vi "End Transaction.vi"(8 "error in (no error)":errorcluster, 11 "SqlMapper in":refnum<class "SqlMapper.lvclass">) -> (0 "error out":errorcluster, 3 "SqlMapper out":refnum<class "SqlMapper.lvclass">)   [LabVIEW 2020, in "ORM.lvlib" / "SqlMapper.lvclass"]
uses:
  SqlMapper.lvclass
  SqlMapper.lvclass/SqlMapper.ctl
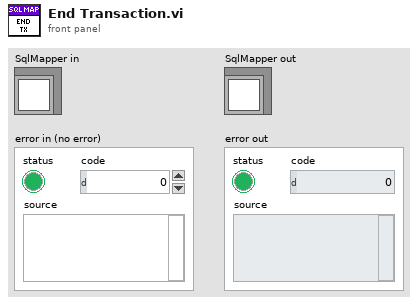
[diagram p1: front panel]
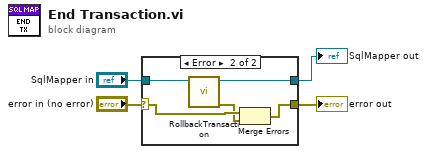
[diagram p0: block diagram]
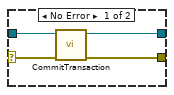
[diagram p2: hidden frame]
diagram:
  n1 = case shown="Error" "error in (no error)" {
    selector: "error in (no error)" -> [w8 w10]
    tunnel: [w7 w11] -> w4
    tunnel: "SqlMapper in" -> [w6 w13]
    tunnel: [w5 w12] -> w3
    frame No Error {
      n2 = call-dynamic "CommitTransaction.vi"("error in (no error)"=w8, "SqlMapper in"=w6) -> ("error out"=w7:errorcluster, "SqlMapper out"=w5:refnum<class "SqlMapper.lvclass">)  [unwired: 8 in]
    }
    frame Error {
      n3 = call-dynamic "RollbackTransaction.vi"("SqlMapper in"=w13) -> ("error out"=w9:errorcluster, "SqlMapper out"=w12:refnum<class "SqlMapper.lvclass">)  [unwired: 9 in]
      n4 = Merge Errors(w10, w9) -> (w11:errorcluster)
    }
  }
  "error out" <- w4
  "SqlMapper out" <- w3
